vi "FRCts20_Backend_Request_GET_reform.vi"(7 "Requests":T1, 8 "error in (no error)":errorcluster, 10 "note data":variant[][](array[variant]), 11 "request data":variant[][](array[variant])) -> (0 "error out":errorcluster, 3 "data string":string)   [LabVIEW 2014, in "FRCts20_Backend_Engine.lvlib"]
doc: "Parses and returns the specific request's data"
uses:
  FRCts20_Backend_Engine.lvlib
  FRCts20_Backend_API/Requests.ctl
  FRCts20_Backend_API/Request.ctl
  FRCts20_Backend_API/ApiReturn.ctl
  FRCts20_Backend_API/FRCts20_Backend_API_Status.ctl
  FRCts20_Backend_API/NotesRoot.ctl
  <vilib>/addons/database/_DB Variant To Data/Database Variant To Data.xnode
  FRCts20_Backend_API/FRCts20_Backend_API.lvlib
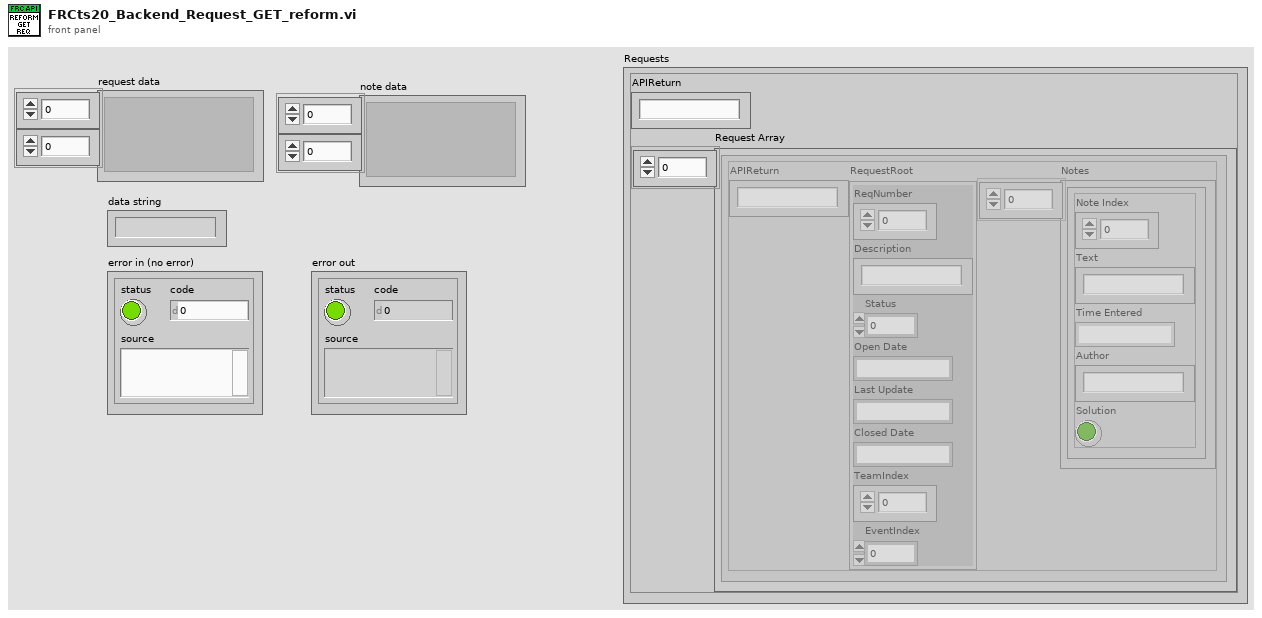
[diagram p1: front panel]
types:
  T1 = typedef "FRCts20_Backend_Engine.lvlib/FRCts20_Backend_API.lvlib/Requests.ctl" = cluster{"APIReturn":string, "Request Array":T2[]}
  T2 = typedef "FRCts20_Backend_Engine.lvlib/FRCts20_Backend_API.lvlib/Request.ctl" = cluster{"APIReturn":T3, "RequestRoot":cluster{"ReqNumber":i32, "Description":string, "Status":T4, "Open Date":string, "Last Update":string, "Closed Date":string, "TeamIndex":i32, "EventIndex":i32}, "Notes":T5}
  T3 = typedef "FRCts20_Backend_Engine.lvlib/FRCts20_Backend_API.lvlib/ApiReturn.ctl" = string
  T4 = typedef "FRCts20_Backend_Engine.lvlib/FRCts20_Backend_API.lvlib/FRCts20_Backend_API_Status.ctl" = i32
  T5 = typedef "FRCts20_Backend_Engine.lvlib/FRCts20_Backend_API.lvlib/NotesRoot.ctl" = cluster{"Note Index":u32, "Text":string, "Time Entered":string, "Author":string, "Solution":bool}[]
  T6 = cluster{"ReqNumber":i32, "Description":string, "Status":T4, "Open Date":string, "Last Update":string, "Closed Date":string, "TeamIndex":i32, "EventIndex":i32}
  T7 = cluster{"ReqNumber":i32, "Description":string, "Status":T4, "Open Date":string, "Last Update":string, "Closed Date":string, "TeamIndex":i32, "EventIndex":i32}[]
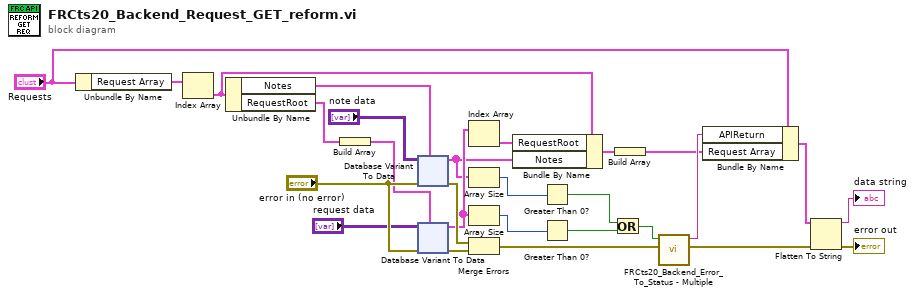
[diagram p0: block diagram]
diagram:
  n1 = Unbundle By Name("Requests") -> ("Request Array"=w14:T2[])
  n2 = Index Array(array=w14) -> (element=w5:T2)  [unwired: 1 in]
  n3 = Unbundle By Name(w5) -> ("Notes"=w8:T5, "RequestRoot"=w7:T6)
  n4 = Build Array(w7) -> (w6:T7)
  n5 = xnode "Database Variant To Data"("database variant"="note data", "error in (no error)"="error in (no error)", "type"=w8) -> ("data"=w3:T5, "error out"=w22:errorcluster)
  n6 = xnode "Database Variant To Data"("database variant"="request data", "error in (no error)"="error in (no error)", "type"=w6) -> ("data"=w18:T7, "error out"=w21:errorcluster)
  n7 = Index Array(array=w18) -> (element=w4:T6)  [unwired: 1 in]
  n8 = Array Size(array=w3) -> (size(s)=w11:i32)
  n9 = Array Size(array=w18) -> (size(s)=w13:i32)
  n10 = Merge Errors(w22, w21) -> (w20:errorcluster)
  n11 = Bundle By Name(cluster=w5, "RequestRoot"=w4, "Notes"=w3) -> (w2:T2)
  n12 = Greater Than 0?(x=w11) -> (x > 0?=w10:bool)
  n13 = Greater Than 0?(x=w13) -> (x > 0?=w12:bool)
  n14 = Or(x=w10, y=w12) -> (x .or. y?=w9:bool)
  n15 = Build Array(w2) -> (w1:T2[])
  n16 = call "FRCts20_Backend_Error_To_Status - Multiple.vi"("error in (no error)"=w20, "rows affected?"=w9) -> ("error out"=w19:errorcluster, "String"=w17:string)  [unwired: 8 in]
  n17 = Bundle By Name(cluster="Requests", "APIReturn"=w17, "Request Array"=w1) -> (w16:T1)
  n18 = Flatten To String(anything=w16, error in (no error)=w19) -> (data string=→"data string":string, error out=→"error out":errorcluster)  [unwired: 2 in, 1 out]
